vi "String to Array.vi"(11 "string":string) -> (3 "Array":string[](array[string]))   [LabVIEW 2018]
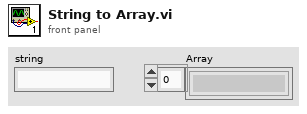
[diagram p1: front panel]
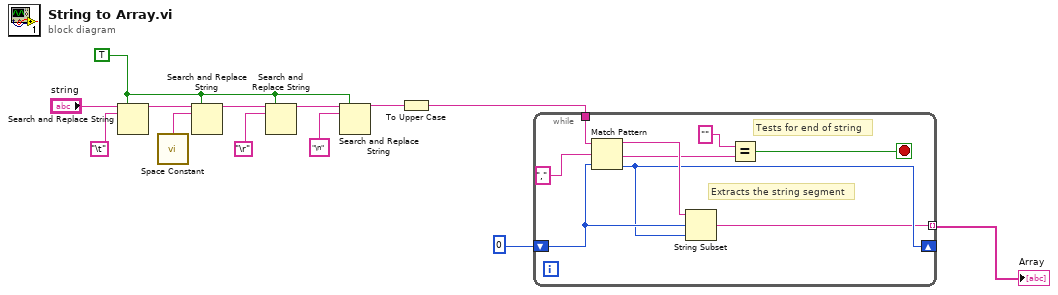
[diagram p0: block diagram]
diagram:
  w4 = TRUE ("replace all? (F)")
  n1 = Search and Replace String(replace all?=w4, input string="string", search string="\t") -> (result string=w9:string)  [unwired: 5 in, 3 out]
  n2 = call <vilib>:"Space Constant.vi"() -> ("String"=w6:string)
  n3 = Search and Replace String(replace all?=w4, input string=w9, search string=w6) -> (result string=w10:string)  [unwired: 5 in, 3 out]
  n4 = Search and Replace String(replace all?=w4, input string=w10, search string="\r") -> (result string=w11:string)  [unwired: 5 in, 3 out]
  n5 = Search and Replace String(replace all?=w4, input string=w11, search string="\n") -> (result string=w3:string)  [unwired: 5 in, 3 out]
  n6 = To Upper Case(1:w3) -> (0:w2:string)
  n7 = while {
    shift-right: [w19] -> _
    shift-left: 0 ("offset past match") -> [w20]
    tunnel: [w18] -> w1 mode=indexing
    tunnel: w2 -> [w14]
    stop <- w15 stop-if-true
    # "Tests for end of string"
    # "Extracts the string segment"
    n8 = Match Pattern(string=w14, regular expression=",", offset (0)=w20) -> (before substring=w21:string, after substring=w17:string, offset past match=w19:i32)  [unwired: 1 out]
    n9 = String Subset(string=w21, offset (0)=w20, length (rest)=w19) -> (substring=w18:string)
    n10 = Equal?(x="", y=w17) -> (x = y?=w15:bool)
  }
  "Array" <- w1
